vi "GLOBAL2.vi"() -> ()   [LabVIEW 2018]
uses:
  GLOBAL DATA INITIALIZE.vi
panel:
  out "Boolean":bool
  out "Gauge":dbl(knob) scale=0.0..100.0
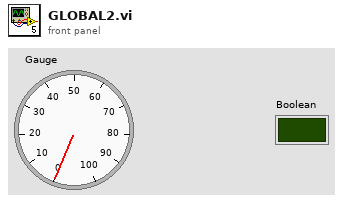
[diagram p1: front panel]
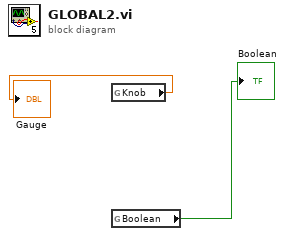
[diagram p0: block diagram]
diagram:
  n1 = global read "GLOBAL DATA INITIALIZE.vi" "Knob"() -> (→"Gauge":dbl)
  n2 = global read "GLOBAL DATA INITIALIZE.vi" "Boolean"() -> (→"Boolean":bool)
